vi "IMAQdx Acquisition Template (Host)-test.vi"() -> ()   [LabVIEW 2016]
uses:
  <vilib>/userdefined/High Color/IMAQdx.ctl
  <vilib>/vision/driver/IMAQdx.llb/IMAQdx Acquisition Mode.ctl
  <vilib>/vision/driver/IMAQdx.llb/IMAQdx Buffer Number Mode.ctl
  <vilib>/FPGAPlugInAG/roboRIO/niLvFpga_Open_roboRIO.vi
  <vilib>/rvi/interface/common/dynamic/niFpgaDynamicAddResources.vi
  <vilib>/FPGAPlugInAG/Dynamic/niLvFpga_Download_Dynamic.vi
  <vilib>/FPGAPlugInAG/Dynamic/niLvFpga_Run_Dynamic.vi
  <vilib>/visionFPGA/Basics/Configure Image Transfer to Target/IMAQ FPGA Configure Image Transfer to Target U32.vi
  <vilib>/Utility/error.llb/Error Cluster From Error Code.vi
  <vilib>/rvi/errors/niLvFpgaAdjustHostInterfaceError.vi
  <vilib>/visionFPGA/Basics/Image Transfer to Target/IMAQ FPGA Image Transfer to Target U32.vi
  <vilib>/rvi/interface/common/niFpgaWaitOnOcc.vi
  <vilib>/FPGAPlugInAG/Dynamic/niLvFpga_Close_Dynamic.vi
  <vilib>/rvi/interface/nirviOpenFPGA/nirviOpenFPGA.xnode
  FPGA Bitfiles/ImageProcessingw_FPGATarget2_ImageProcessingw_ZcF2hsHpmf8.lvbitx
  <vilib>/rvi/interface/nirviMethod/nirviMethod.xnode
  <vilib>/rvi/interface/nirviReadWriteControl/nirviReadWriteControl.xnode
  <vilib>/rvi/interface/nirviCloseFPGA/nirviCloseFPGA.xnode
  <vilib>/vision/driver/NI_Vision_Acquisition_Software.lvlib
  <resource>/objmgr/imaqdx.rc
  <vilib>/visionFPGA/NI_VDM_FPGA_Basics.lvlib
  <vilib>/rvi/interface/Simulation/niFpgaSimulationCallBeginRW.vi
  <vilib>/rvi/errors/niLvFpgaMergeErrorWithErrorCode.vi
  <vilib>/FPGAPlugInAG/Dynamic/niLvFpga_ReadFifo_Dynamic.vi
  <vilib>/FPGAPlugInAG/Dynamic/niLvFpga_ConfigureFifo_Dynamic.vi
  <vilib>/FPGAPlugInAG/Dynamic/niLvFpga_StartFifo_Dynamic.vi
  NiFpgaLv.dll
panel:
  out "OriImage Err out":errorcluster
  out "Image":T1(plugin-control)
  out "Count":i32
  out "error out 2":errorcluster
  in  "Camera":T2
  out "Error Out":errorcluster
  in  "Stop":bool
  # "Overview: Demonstrates how to acquire an image from a camera using the IMAQdx API, transfer the image to a FPGA target for processing, and retrieve the processed image for display or further processing on the host.\nRequirements:\n- LabVIEW FPGA\n- Vision Acquisition Software\n- Vision Development Module\nInstructions:\n1. Select a Camera\n2. Run the VI."
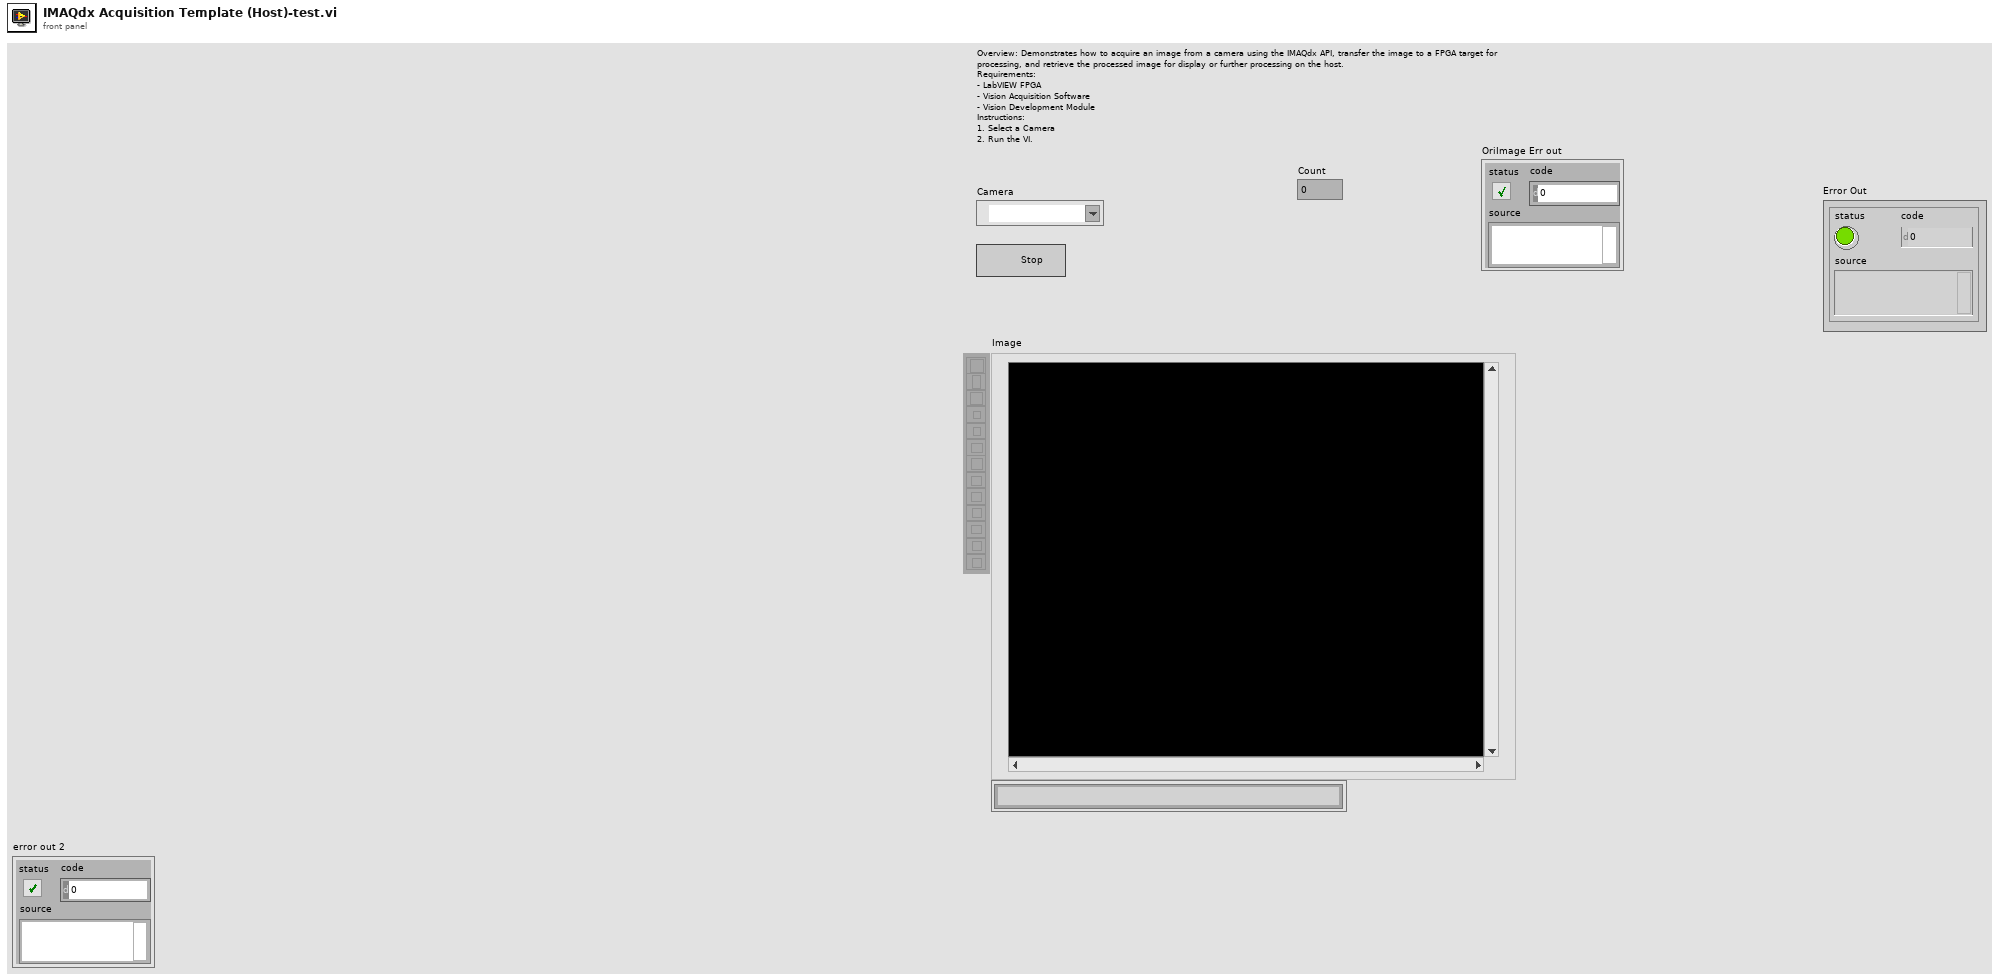
[diagram p1: front panel]
types:
  T1 = typedef "IMAQ Image.ctl" = refnum<image>
  T2 = typedef "IMAQdx.ctl" = refnum<k21>
  T3 = typedef "Image Type" = u32
  T4 = typedef "NI_Vision_Acquisition_Software.lvlib/IMAQdx Acquisition Mode.ctl" = enum32{"One Shot", "Continuous"}
  T5 = typedef "NI_Vision_Acquisition_Software.lvlib/IMAQdx Buffer Number Mode.ctl" = enum32{"Next", "Last", "Buffer Number", "Every", "Last New"}
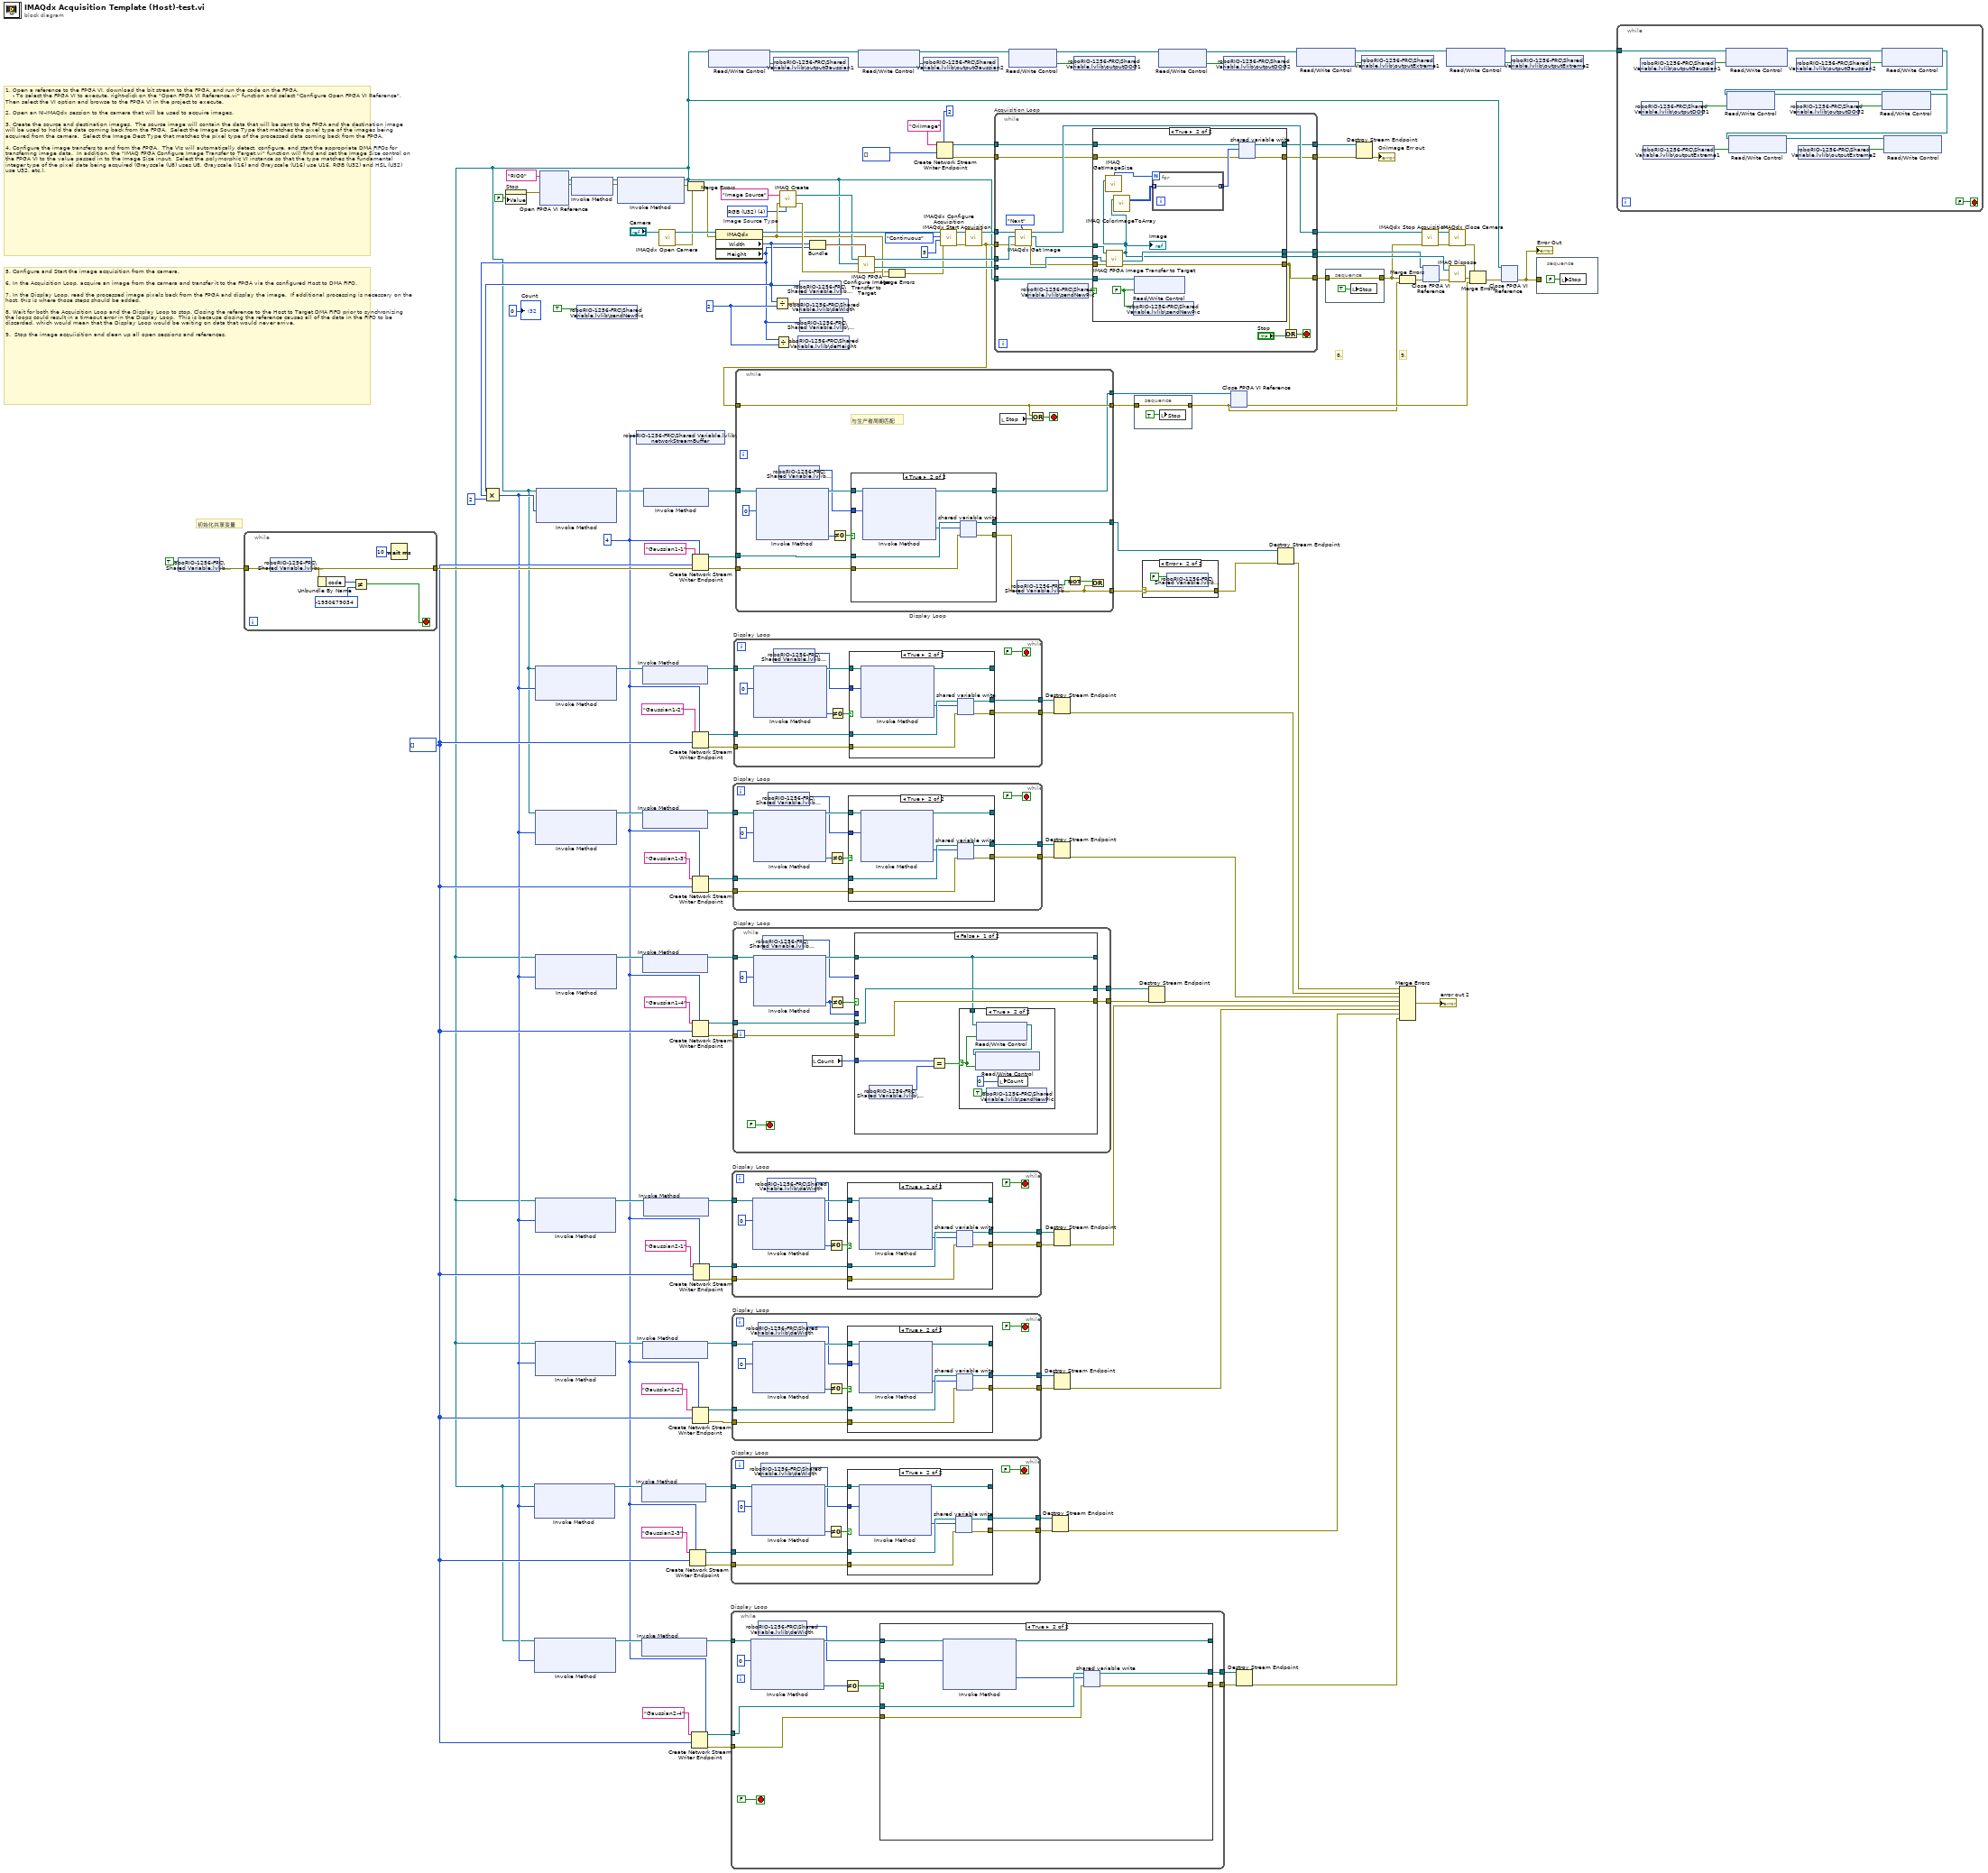
[diagram p0: block diagram]
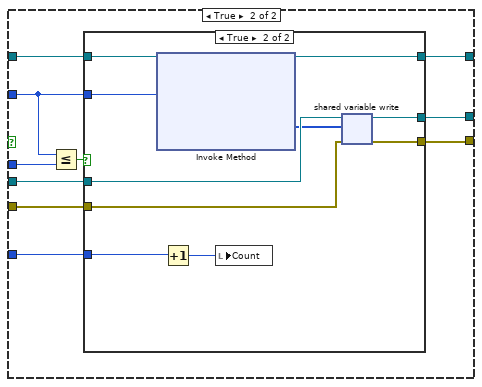
[diagram p6: hidden frame]
diagram:
  w16 = u32 2 ("y")
  w28 = i32[] []
  w25 = 4 ("writer buffer size")
  w110 = T3 4 items=["Grayscale (U8)", "Grayscale (I16)", "Grayscale (SGL)", "Complex (CSG)", "RGB (U32)", "HSL (U32)", "RGB (U64)", "Grayscale (U16)"]  # Image Source Type
  # "初始化共享变量"
  # "5. Configure and Start the image acquisition from the camera.\n\n6. In the Acquisition Loop, acquire an image from the camera and transfer it to the FPGA via the configured Host to DMA FIFO.\n\n7. In the Display Loop, read the processed image pixels back from the FPGA and display the image.  If additional processing is necessary on the host, this is where those steps should be added.\n\n8. Wait for both the Acquisition Loop and the Display Loop to stop. Closing the reference to the Host to Target DMA FIFO prior to synchronizing the loops could result in a timeout error in the Display Loop.  This is because closing the reference causes all of the data in the FIFO to be discarded, which would mean that the Display Loop would be waiting on data that would never arrive.\n\n9.  Stop the image acquiisition and clean up all open sessions and references."
  # "1. Open a reference to the FPGA VI, download the bit stream to the FPGA, and run the code on the FPGA.\n    - To select the FPGA VI to execute, right-click on the \"Open FPGA VI Reference.vi\" function and select \"Configure Open FPGA VI Reference\".  Then select the VI option and browse to the FPGA VI in the project to execute.\n\n2. Open an NI-IMAQdx session to the camera that will be used to acquire images.\n\n3. Create the source and destination images.  The source image will contain the data that will be sent to the FPGA and the destination image will be used to hold the data coming back from the FPGA.  Select the Image Source Type that matches the pixel type of the images being acquired from the camera.  Select the Image Dest Type that matches the pixel type of the processed data coming back from the FPGA.\n\n4. Configure the image transfers to and from the FPGA.  The VIs will automatically detect, configure, and start the appropriate DMA FIFOs for transferring image data.  In addition, the \"IMAQ FPGA Configure Image Transfer to Target.vi\" function will find and set the Image Size control on the FPGA VI to the value passed in to the Image Size input.  Select the polymorphic VI instance so that the type matches the fundamental integer type of the pixel data being acquired (Grayscale (U8) uses U8, Grayscale (I16) and Grayscale (U16) use U16, RGB (U32) and HSL (U32) use U32, etc.)."
  # "9."
  # "8."
  n1 = shared-variable "roboRIO-1256-FRC\\Shared Variable.lvlib\\Active"(TRUE ("Active?")) -> (error out=w96:errorcluster)  [unwired: 1 in]
  n2 = while {
    tunnel: w96 -> [w153]
    tunnel: [w150] -> w95
    stop <- w149 stop-if-true
    n3 = shared-variable "roboRIO-1256-FRC\\Shared Variable.lvlib\\Active"(error in=w153) -> (error out=w150:errorcluster)  [unwired: 1 out]
    n4 = Unbundle By Name(w150) -> ("code"=w152:i32)
    n5 = Not Equal?(x=w152, y=-1950679034) -> (x != y?=w149:bool)
    n6 = Wait (ms)(milliseconds to wait=u32 10) -> ()  [unwired: 1 out]
  }
  n7 = property on="Stop" class="Bool (strict)"("Value"=FALSE ("Stop")) -> (error out=w145:errorcluster)  [unwired: 2 in, 1 out]
  n8 = xnode "Open FPGA VI Reference"("error in"=w145, "resource name"=tag "RIO0") -> ("FPGA VI Reference Out"=w141:refnum<k20>, "error out"=w142:errorcluster)
  n9 = xnode "Invoke Method"("FPGA VI Reference In"=w141, "error in"=w142) -> ("FPGA VI Reference Out"=w144:refnum<k20>, "error out"=w143:errorcluster)
  n10 = shared-variable "roboRIO-1256-FRC\\Shared Variable.lvlib\\sendNewPic"(TRUE) -> ()  [unwired: 1 in, 1 out]
  n11 = xnode "Invoke Method"("FPGA VI Reference In"=w144, "error in"=w143) -> ("FPGA VI Reference Out"=w2:refnum<k20>, "error out"=w130:errorcluster)  [unwired: 1 in]
  n12 = shared-variable "roboRIO-1256-FRC\\Shared Variable.lvlib\\networkStreamBuffer"(w25) -> ()  [unwired: 1 in, 1 out]
  n13 = call <vilib>:"IMAQdx Open Camera.vi"("Session In"="Camera") -> ("error out"=w115:errorcluster, "Session Out"=w116:T2)  [unwired: 9 in]
  n14 = Merge Errors(w130, w115) -> (w114:errorcluster)
  n15 = Create Network Stream Writer Endpoint(7:w25, 9:w28, 11:"Gaussian2-3" ("writer name")) -> (0:w32:errorcluster, 3:w31:refnum<k21>)  [unwired: 4 in]
  n16 = Create Network Stream Writer Endpoint(7:w25, 9:w28, 11:"Gaussian2-4" ("writer name")) -> (0:w57:errorcluster, 3:w58:refnum<k21>)  [unwired: 4 in]
  n17 = Create Network Stream Writer Endpoint(7:w25, 9:w28, 11:"Gaussian2-2" ("writer name")) -> (0:w39:errorcluster, 3:w40:refnum<k21>)  [unwired: 4 in]
  n18 = Create Network Stream Writer Endpoint(7:w25, 8:w95, 9:w28, 11:"Gaussian1-1" ("writer name")) -> (0:w91:errorcluster, 3:w90:refnum<k21>)  [unwired: 3 in]
  n19 = Create Network Stream Writer Endpoint(7:w25, 9:w28, 11:"Gaussian1-2" ("writer name")) -> (0:w72:errorcluster, 3:w73:refnum<k21>)  [unwired: 4 in]
  n20 = Create Network Stream Writer Endpoint(7:w25, 9:w28, 11:"Gaussian1-3" ("writer name")) -> (0:w67:errorcluster, 3:w66:refnum<k21>)  [unwired: 4 in]
  n21 = Create Network Stream Writer Endpoint(7:w25, 9:w28, 11:"Gaussian1-4" ("writer name")) -> (0:w51:errorcluster, 3:w52:refnum<k21>)  [unwired: 4 in]
  n22 = Create Network Stream Writer Endpoint(7:w25, 9:w28, 11:"Gaussian2-1" ("writer name")) -> (0:w46:errorcluster, 3:w45:refnum<k21>)  [unwired: 4 in]
  n23 = xnode "Read/Write Control"("FPGA VI Reference In"=w2) -> ("FPGA VI Reference Out"=w11:refnum<k20>, "outputGaussian1"=w13:bool)  [unwired: 1 in, 1 out]
  n24 = property class="IMAQdx"(reference=w116, error in=w114) -> (reference out=w123:T2, error out=w111:errorcluster, "Width"=w18:u32, "Height"=w15:u32)
  n25 = Compound Arithmetic op=MULTIPLY(w18, w15, u32 2 ("value")) -> (w24:u32)
  n26 = xnode "Invoke Method"("FPGA VI Reference In"=w2, "Requested Depth"=w24) -> ("FPGA VI Reference Out"=w33:refnum<k20>)  [unwired: 1 in, 2 out]
  n27 = xnode "Invoke Method"("FPGA VI Reference In"=w2, "Requested Depth"=w24) -> ("FPGA VI Reference Out"=w56:refnum<k20>)  [unwired: 1 in, 2 out]
  n28 = xnode "Invoke Method"("FPGA VI Reference In"=w2, "Requested Depth"=w24) -> ("FPGA VI Reference Out"=w27:refnum<k20>)  [unwired: 1 in, 2 out]
  n29 = xnode "Invoke Method"("FPGA VI Reference In"=w2, "Requested Depth"=w24) -> ("FPGA VI Reference Out"=w38:refnum<k20>)  [unwired: 1 in, 2 out]
  n30 = xnode "Invoke Method"("FPGA VI Reference In"=w2, "Requested Depth"=w24) -> ("FPGA VI Reference Out"=w71:refnum<k20>)  [unwired: 1 in, 2 out]
  n31 = xnode "Invoke Method"("FPGA VI Reference In"=w2, "Requested Depth"=w24) -> ("FPGA VI Reference Out"=w68:refnum<k20>)  [unwired: 1 in, 2 out]
  n32 = xnode "Invoke Method"("FPGA VI Reference In"=w2, "Requested Depth"=w24) -> ("FPGA VI Reference Out"=w50:refnum<k20>)  [unwired: 1 in, 2 out]
  n33 = xnode "Invoke Method"("FPGA VI Reference In"=w2, "Requested Depth"=w24) -> ("FPGA VI Reference Out"=w100:refnum<k20>)  [unwired: 1 in, 2 out]
  n34 = xnode "Invoke Method"("FPGA VI Reference In"=w33) -> ("FPGA VI Reference Out"=w34:refnum<k20>)  [unwired: 1 in, 1 out]
  n35 = xnode "Invoke Method"("FPGA VI Reference In"=w56) -> ("FPGA VI Reference Out"=w55:refnum<k20>)  [unwired: 1 in, 1 out]
  n36 = xnode "Invoke Method"("FPGA VI Reference In"=w38) -> ("FPGA VI Reference Out"=w37:refnum<k20>)  [unwired: 1 in, 1 out]
  n37 = xnode "Invoke Method"("FPGA VI Reference In"=w71) -> ("FPGA VI Reference Out"=w70:refnum<k20>)  [unwired: 1 in, 1 out]
  n38 = xnode "Invoke Method"("FPGA VI Reference In"=w68) -> ("FPGA VI Reference Out"=w69:refnum<k20>)  [unwired: 1 in, 1 out]
  n39 = xnode "Invoke Method"("FPGA VI Reference In"=w50) -> ("FPGA VI Reference Out"=w49:refnum<k20>)  [unwired: 1 in, 1 out]
  n40 = xnode "Invoke Method"("FPGA VI Reference In"=w100) -> ("FPGA VI Reference Out"=w99:refnum<k20>)  [unwired: 1 in, 1 out]
  n41 = xnode "Invoke Method"("FPGA VI Reference In"=w27) -> ("FPGA VI Reference Out"=w26:refnum<k20>)  [unwired: 1 in, 1 out]
  n42 = while "Display Loop" {
    tunnel: [w164] -> w61
    tunnel: w57 -> [w163]
    tunnel: w58 -> [w162]
    tunnel: [w157] -> w60
    tunnel: w55 -> [w156]
    stop <- FALSE stop-if-true
    n43 = xnode "Invoke Method"("FPGA VI Reference In"=w156, "Number of Elements"=u32 0) -> ("FPGA VI Reference Out"=w159:refnum<k20>, "Elements Remaining"=w154:u32)  [unwired: 2 in, 2 out]
    n44 = shared-variable "roboRIO-1256-FRC\\Shared Variable.lvlib\\deWidth"() -> (w155:u16)  [unwired: 1 in, 1 out]
    n45 = Not Equal To 0?(x=w154) -> (x != 0?=w161:bool)
    n46 = case shown="True" w161 {
      tunnel: w159 -> [w165 w175]
      tunnel: [w167 w174] -> w164
      tunnel: w163 -> [w166 w173]
      tunnel: w162 -> [w167 w172]
      tunnel: [w166 w171] -> w157
      tunnel: [w165 w170] -> _
      tunnel: w155 -> [_ w169]
      frame False {
      }
      frame True {
        n47 = xnode "Invoke Method"("FPGA VI Reference In"=w175, "Number of Elements"=w169) -> ("FPGA VI Reference Out"=w170:refnum<k20>, "Data"=w168:u8[])  [unwired: 2 in, 2 out]
        n48 = shared-variable-write(w172, w173, w168) -> (w174:refnum<k21>, w171:errorcluster)  [unwired: 1 in, 1 out]
      }
    }
  }
  n49 = while "Display Loop" {
    tunnel: [w186] -> w29
    tunnel: w32 -> [w185]
    tunnel: w31 -> [w184]
    tunnel: [w178] -> w30
    tunnel: w34 -> [w177]
    stop <- FALSE stop-if-true
    (unwired) u32 640 ("Number of Elements")
    n50 = xnode "Invoke Method"("FPGA VI Reference In"=w177, "Number of Elements"=u32 0) -> ("FPGA VI Reference Out"=w180:refnum<k20>, "Elements Remaining"=w181:u32)  [unwired: 2 in, 2 out]
    n51 = shared-variable "roboRIO-1256-FRC\\Shared Variable.lvlib\\deWidth"() -> (w176:u16)  [unwired: 1 in, 1 out]
    n52 = Not Equal To 0?(x=w181) -> (x != 0?=w183:bool)
    n53 = case shown="True" w183 {
      tunnel: w180 -> [w187 w197]
      tunnel: [w189 w196] -> w186
      tunnel: w185 -> [w188 w195]
      tunnel: w184 -> [w189 w194]
      tunnel: [w188 w193] -> w178
      tunnel: [w187 w191] -> _
      tunnel: w176 -> [_ w190]
      frame False {
      }
      frame True {
        n54 = xnode "Invoke Method"("FPGA VI Reference In"=w197, "Number of Elements"=w190) -> ("FPGA VI Reference Out"=w191:refnum<k20>, "Data"=w192:u8[])  [unwired: 2 in, 2 out]
        n55 = shared-variable-write(w194, w195, w192) -> (w196:refnum<k21>, w193:errorcluster)  [unwired: 1 in, 1 out]
      }
    }
  }
  n56 = while "Display Loop" {
    tunnel: [w208] -> w43
    tunnel: w46 -> [w207]
    tunnel: w45 -> [w206]
    tunnel: [w200] -> w44
    tunnel: w26 -> [w199]
    stop <- FALSE stop-if-true
    (unwired) u32 640 ("Number of Elements")
    n57 = xnode "Invoke Method"("FPGA VI Reference In"=w199, "Number of Elements"=u32 0) -> ("FPGA VI Reference Out"=w202:refnum<k20>, "Elements Remaining"=w203:u32)  [unwired: 2 in, 2 out]
    n58 = shared-variable "roboRIO-1256-FRC\\Shared Variable.lvlib\\deWidth"() -> (w198:u16)  [unwired: 1 in, 1 out]
    n59 = Not Equal To 0?(x=w203) -> (x != 0?=w205:bool)
    n60 = case shown="True" w205 {
      tunnel: w202 -> [w209 w219]
      tunnel: [w211 w218] -> w208
      tunnel: w207 -> [w210 w217]
      tunnel: w206 -> [w211 w216]
      tunnel: [w210 w215] -> w200
      tunnel: [w209 w213] -> _
      tunnel: w198 -> [_ w212]
      frame False {
      }
      frame True {
        n61 = xnode "Invoke Method"("FPGA VI Reference In"=w219, "Number of Elements"=w212) -> ("FPGA VI Reference Out"=w213:refnum<k20>, "Data"=w214:u8[])  [unwired: 2 in, 2 out]
        n62 = shared-variable-write(w216, w217, w214) -> (w218:refnum<k21>, w215:errorcluster)  [unwired: 1 in, 1 out]
      }
    }
  }
  n63 = while "Display Loop" {
    tunnel: [w230] -> w42
    tunnel: w39 -> [w229]
    tunnel: w40 -> [w228]
    tunnel: [w222] -> w41
    tunnel: w37 -> [w221]
    stop <- FALSE stop-if-true
    (unwired) u32 640 ("Number of Elements")
    n64 = xnode "Invoke Method"("FPGA VI Reference In"=w221, "Number of Elements"=u32 0) -> ("FPGA VI Reference Out"=w224:refnum<k20>, "Elements Remaining"=w225:u32)  [unwired: 2 in, 2 out]
    n65 = shared-variable "roboRIO-1256-FRC\\Shared Variable.lvlib\\deWidth"() -> (w220:u16)  [unwired: 1 in, 1 out]
    n66 = Not Equal To 0?(x=w225) -> (x != 0?=w227:bool)
    n67 = case shown="True" w227 {
      tunnel: w224 -> [w231 w241]
      tunnel: [w233 w240] -> w230
      tunnel: w229 -> [w232 w239]
      tunnel: w228 -> [w233 w238]
      tunnel: [w232 w237] -> w222
      tunnel: [w231 w235] -> _
      tunnel: w220 -> [_ w234]
      frame False {
      }
      frame True {
        n68 = xnode "Invoke Method"("FPGA VI Reference In"=w241, "Number of Elements"=w234) -> ("FPGA VI Reference Out"=w235:refnum<k20>, "Data"=w236:u8[])  [unwired: 2 in, 2 out]
        n69 = shared-variable-write(w238, w239, w236) -> (w240:refnum<k21>, w237:errorcluster)  [unwired: 1 in, 1 out]
      }
    }
  }
  n70 = while "Display Loop" {
    tunnel: [w252] -> w63
    tunnel: w67 -> [w251]
    tunnel: w66 -> [w250]
    tunnel: [w244] -> w64
    tunnel: w69 -> [w243]
    stop <- FALSE stop-if-true
    (unwired) u32 640 ("Number of Elements")
    n71 = xnode "Invoke Method"("FPGA VI Reference In"=w243, "Number of Elements"=u32 0) -> ("FPGA VI Reference Out"=w246:refnum<k20>, "Elements Remaining"=w247:u32)  [unwired: 2 in, 2 out]
    n72 = shared-variable "roboRIO-1256-FRC\\Shared Variable.lvlib\\Width"() -> (w242:u16)  [unwired: 1 in, 1 out]
    n73 = Not Equal To 0?(x=w247) -> (x != 0?=w249:bool)
    n74 = case shown="True" w249 {
      tunnel: w246 -> [w253 w263]
      tunnel: [w255 w262] -> w252
      tunnel: w251 -> [w254 w261]
      tunnel: w250 -> [w255 w260]
      tunnel: [w254 w259] -> w244
      tunnel: [w253 w257] -> _
      tunnel: w242 -> [_ w256]
      frame False {
      }
      frame True {
        n75 = xnode "Invoke Method"("FPGA VI Reference In"=w263, "Number of Elements"=w256) -> ("FPGA VI Reference Out"=w257:refnum<k20>, "Data"=w258:u8[])  [unwired: 2 in, 2 out]
        n76 = shared-variable-write(w260, w261, w258) -> (w262:refnum<k21>, w259:errorcluster)  [unwired: 1 in, 1 out]
      }
    }
  }
  n77 = while "Display Loop" {
    tunnel: [w275] -> w54
    tunnel: w51 -> [w274]
    tunnel: w52 -> [w273]
    tunnel: [w268] -> w53
    tunnel: w49 -> [w267]
    stop <- FALSE stop-if-true
    n78 = xnode "Invoke Method"("FPGA VI Reference In"=w267, "Number of Elements"=u32 0) -> ("FPGA VI Reference Out"=w270:refnum<k20>, "Elements Remaining"=w264:u32)  [unwired: 2 in, 2 out]
    n79 = shared-variable "roboRIO-1256-FRC\\Shared Variable.lvlib\\Width"() -> (w266:u16)  [unwired: 1 in, 1 out]
    n80 = local read "Count"() -> (w265:i32)
    n81 = Not Equal To 0?(x=w264) -> (x != 0?=w272:bool)
    n82 = case shown="False" w272 {
      tunnel: w270 -> [w276 w296]
      tunnel: [w281 w295] -> w275
      tunnel: w274 -> [w280 w294]
      tunnel: w273 -> [w281 w293]
      tunnel: [w280 w292] -> w268
      tunnel: [w276 w291] -> _
      tunnel: w266 -> [_ w288]
      tunnel: w265 -> [w278 w290]
      tunnel: w264 -> [_ w287]
      frame False {
        n83 = shared-variable "roboRIO-1256-FRC\\Shared Variable.lvlib\\Height"() -> (w277:u16)  [unwired: 1 in, 1 out]
        n84 = Equal?(x=w278, y=w277) -> (x = y?=w279:bool)
        n85 = case shown="True" w279 {
          selector: w279 -> [_ w283]
          tunnel: w276 -> [_ w286]
          frame False {
          }
          frame True {
            n86 = xnode "Read/Write Control"("FPGA VI Reference In"=w286, "StartOfImage"=w283) -> ("FPGA VI Reference Out"=w285:refnum<k20>)  [unwired: 1 in, 1 out]
            n87 = xnode "Read/Write Control"("FPGA VI Reference In"=w285, "Ready For Output"=w283) -> ()  [unwired: 1 in, 2 out]
            n88 = shared-variable "roboRIO-1256-FRC\\Shared Variable.lvlib\\sendNewPic"(TRUE ("sendNewPic")) -> ()  [unwired: 1 in, 1 out]
            n89 = local write "Count"(0) -> ()
          }
        }
      }
      frame True {
        n90 = Less Or Equal?(x=w288, y=w287) -> (x <= y?=w289:bool)
        n91 = case shown="True" w289 {
          tunnel: w296 -> [w299 w309]
          tunnel: [w298 w308] -> w295
          tunnel: w294 -> [w297 w307]
          tunnel: w293 -> [w298 w306]
          tunnel: [w297 w305] -> w292
          tunnel: [w299 w303] -> w291
          tunnel: w288 -> [_ w302]
          tunnel: w290 -> [_ w301]
          frame False {
          }
          frame True {
            n92 = xnode "Invoke Method"("FPGA VI Reference In"=w309, "Number of Elements"=w302) -> ("FPGA VI Reference Out"=w303:refnum<k20>, "Data"=w304:u8[])  [unwired: 2 in, 2 out]
            n93 = Increment(x=w301) -> (x+1=w300:i32)
            n94 = local write "Count"(w300) -> ()
            n95 = shared-variable-write(w306, w307, w304) -> (w308:refnum<k21>, w305:errorcluster)  [unwired: 1 in, 1 out]
          }
        }
      }
    }
  }
  n96 = while "Display Loop" {
    tunnel: [w320] -> w80
    tunnel: w72 -> [w319]
    tunnel: w73 -> [w318]
    tunnel: [w312] -> w79
    tunnel: w70 -> [w311]
    stop <- FALSE stop-if-true
    (unwired) u32 640 ("Number of Elements")
    n97 = xnode "Invoke Method"("FPGA VI Reference In"=w311, "Number of Elements"=u32 0) -> ("FPGA VI Reference Out"=w314:refnum<k20>, "Elements Remaining"=w315:u32)  [unwired: 2 in, 2 out]
    n98 = shared-variable "roboRIO-1256-FRC\\Shared Variable.lvlib\\Width"() -> (w310:u16)  [unwired: 1 in, 1 out]
    n99 = Not Equal To 0?(x=w315) -> (x != 0?=w317:bool)
    n100 = case shown="True" w317 {
      tunnel: w314 -> [w321 w331]
      tunnel: [w323 w330] -> w320
      tunnel: w319 -> [w322 w329]
      tunnel: w318 -> [w323 w328]
      tunnel: [w322 w327] -> w312
      tunnel: [w321 w325] -> _
      tunnel: w310 -> [_ w324]
      frame False {
      }
      frame True {
        n101 = xnode "Invoke Method"("FPGA VI Reference In"=w331, "Number of Elements"=w324) -> ("FPGA VI Reference Out"=w325:refnum<k20>, "Data"=w326:u8[])  [unwired: 2 in, 2 out]
        n102 = shared-variable-write(w328, w329, w326) -> (w330:refnum<k21>, w327:errorcluster)  [unwired: 1 in, 1 out]
      }
    }
  }
  n103 = shared-variable "roboRIO-1256-FRC\\Shared Variable.lvlib\\outputGaussian1"(w13) -> ()  [unwired: 1 in, 1 out]
  n104 = Divide(x=w18, y=w16) -> (x/y=w17:dbl)
  n105 = Divide(x=w15, y=w16) -> (x/y=w14:dbl)
  n106 = call "IMAQ Create"("Image Name"="Image Source", "Image Type"=w110, "error in (no error)"=w111) -> ("New Image"=w121:T1, "error out"=w129:errorcluster)  [unwired: 2 in]
  n107 = shared-variable "roboRIO-1256-FRC\\Shared Variable.lvlib\\deHeight"(w14) -> ()  [unwired: 1 in, 1 out]
  n108 = shared-variable "roboRIO-1256-FRC\\Shared Variable.lvlib\\Width"(w18) -> ()  [unwired: 1 in, 1 out]
  n109 = shared-variable "roboRIO-1256-FRC\\Shared Variable.lvlib\\deWidth"(w17) -> ()  [unwired: 1 in, 1 out]
  n110 = shared-variable "roboRIO-1256-FRC\\Shared Variable.lvlib\\Height"(w15) -> ()  [unwired: 1 in, 1 out]
  n111 = Bundle("Width"=w18, "Height"=w15) -> (w128:cluster{"Width":u32, "Height":u32})  [unwired: 1 in]
  n112 = xnode "Read/Write Control"("FPGA VI Reference In"=w11) -> ("FPGA VI Reference Out"=w7:refnum<k20>, "outputGaussian2"=w12:bool)  [unwired: 1 in, 1 out]
  n113 = call-poly <vilib>:"IMAQ FPGA Configure Image Transfer to Target.vi"("Image Size"=w128, "error in (no error)"=w129, "FPGA VI Reference In"=w2, "Image"=w121) -> ("error out"=w104:errorcluster, "DMA FIFO Reference Out"=w139:refnum<k20>, "Image Out"=w140:T1)  [unwired: 4 in, 1 out]
  n114 = Merge Errors(w104, w111) -> (w103:errorcluster)
  n115 = shared-variable "roboRIO-1256-FRC\\Shared Variable.lvlib\\outputGaussian2"(w12) -> ()  [unwired: 1 in, 1 out]
  n116 = Create Network Stream Writer Endpoint(7:2 ("writer buffer size"), 9:i32[] [], 11:"OriImage" ("writer name")) -> (0:w84:errorcluster, 3:w85:refnum<k21>)  [unwired: 4 in]
  n117 = call <vilib>:"IMAQdx Configure Acquisition.vi"("error in"=w103, "Number of Buffers"=u32 5, "Continuous?"=IMAQdx_Acquisition_Mode."Continuous", "Session In"=w123) -> ("error out"=w126:errorcluster, "Session Out"=w127:T2)  [unwired: 6 in]
  n118 = call <vilib>:"IMAQdx Start Acquisition.vi"("error in"=w126, "Session In"=w127) -> ("error out"=w102:errorcluster, "Session Out"=w122:T2)  [unwired: 8 in]
  n119 = while "Display Loop" {
    tunnel: w102 -> [w347]
    tunnel: [w335] -> w136
    tunnel: [w347] -> w135
    tunnel: w99 -> [w336]
    tunnel: [w345] -> w93
    tunnel: [w344] -> w92
    tunnel: w91 -> [w343]
    tunnel: w90 -> [w342]
    stop <- w348 stop-if-true
    (unwired) u32 640 ("Number of Elements")
    # "与生产者周期匹配"
    n120 = xnode "Invoke Method"("FPGA VI Reference In"=w336, "Number of Elements"=u32 0) -> ("FPGA VI Reference Out"=w333:refnum<k20>, "Elements Remaining"=w334:u32)  [unwired: 2 in, 2 out]
    n121 = shared-variable "roboRIO-1256-FRC\\Shared Variable.lvlib\\Width"() -> (w332:u16)  [unwired: 1 in, 1 out]
    n122 = Not Equal To 0?(x=w334) -> (x != 0?=w338:bool)
    n123 = case shown="True" w338 {
      tunnel: w333 -> [w349 w359]
      tunnel: [w351 w358] -> w344
      tunnel: w343 -> [w350 w357]
      tunnel: w342 -> [w351 w356]
      tunnel: [w350 w355] -> w341
      tunnel: [w349 w353] -> w335
      tunnel: w332 -> [_ w352]
      frame False {
      }
      frame True {
        n124 = xnode "Invoke Method"("FPGA VI Reference In"=w359, "Number of Elements"=w352) -> ("FPGA VI Reference Out"=w353:refnum<k20>, "Data"=w354:u8[])  [unwired: 2 in, 2 out]
        n125 = shared-variable-write(w356, w357, w354) -> (w358:refnum<k21>, w355:errorcluster)  [unwired: 1 in, 1 out]
      }
    }
    n126 = local read "Stop"() -> (w346:bool)
    n127 = shared-variable "roboRIO-1256-FRC\\Shared Variable.lvlib\\Active"(error in=w341) -> (w339:bool, error out=w345:errorcluster)
    n128 = Or(x=w347, y=w346) -> (x .or. y?=w348:bool)
    n129 = Not(x=w339) -> (.not. x?=w340:bool)
    n130 = Or(x=w340, y=w345) -> ()  [unwired: 1 out]
  }
  n131 = while "Acquisition Loop" {
    tunnel: [w369] -> w108
    tunnel: w140 -> [w374]
    tunnel: w139 -> [w371]
    tunnel: [w370] -> w109
    tunnel: [w367] -> w138
    tunnel: w122 -> [w375]
    tunnel: [w373] -> w118
    tunnel: w102 -> [w372]
    tunnel: w2 -> [w365]
    tunnel: w85 -> [w364]
    tunnel: w84 -> [w363]
    tunnel: [w362] -> w83
    tunnel: [w361] -> w82
    stop <- w377 stop-if-true
    n132 = call <vilib>:"IMAQdx Get Image.vi"("Buffer Number Mode (Next)"=IMAQdx_Buffer_Number_Mode."Next", "error in"=w372, "Image In"=w374, "Session In"=w375) -> ("error out"=w366:errorcluster, "Image Out"=w368:T1, "Session Out"=w373:T2)  [unwired: 4 in, 1 out]
    n133 = shared-variable "roboRIO-1256-FRC\\Shared Variable.lvlib\\sendNewPic"() -> (w360:bool)  [unwired: 1 in, 1 out]
    n134 = case shown="True" w360 {
      tunnel: w371 -> [w383 w398]
      tunnel: [w383 w394] -> w370
      tunnel: [w382 w395] -> w369
      tunnel: w368 -> [w381 w397]
      tunnel: [w381 w389] -> w367
      tunnel: w366 -> [w382 w396]
      tunnel: w365 -> [_ w392]
      tunnel: w364 -> [w380 w387]
      tunnel: w363 -> [w379 w386]
      tunnel: [w380 w385] -> w362
      tunnel: [w379 w384] -> w361
      frame False {
      }
      frame True {
        w393 = FALSE ("EndOfImage")
        n135 = call-poly <vilib>:"IMAQ FPGA Image Transfer to Target.vi"("error in (no error)"=w396, "DMA FIFO Reference In"=w398, "Image"=w397) -> ("error out"=w395:errorcluster, "DMA FIFO Reference Out"=w394:refnum<k20>, "Image Out"=w389:T1)  [unwired: 6 in]
        "Image" <- w389
        n136 = call "IMAQ GetImageSize"("Image"=w389) -> ("X Resolution"=w391:i32)  [unwired: 3 in, 2 out]
        n137 = call "IMAQ ColorImageToArray"("Image"=w389) -> ("Image Pixels (U32)"=w390:u32[][])  [unwired: 3 in, 2 out]
        n138 = shared-variable "roboRIO-1256-FRC\\Shared Variable.lvlib\\sendNewPic"(w393) -> ()  [unwired: 1 in, 1 out]
        n139 = xnode "Read/Write Control"("FPGA VI Reference In"=w392, "StartOfImage"=w393) -> ()  [unwired: 1 in, 2 out]
        n140 = for {
          N: w391 -> [_]
          tunnel: w390 -> [w399] mode=indexing
          tunnel: [w399] -> w388 mode=concatenating
        }
        n141 = shared-variable-write(w387, w386, w388) -> (w385:refnum<k21>, w384:errorcluster)  [unwired: 1 in, 1 out]
      }
    }
    n142 = Or(x=w369, y="Stop") -> (x .or. y?=w377:bool)
  }
  n143 = xnode "Read/Write Control"("FPGA VI Reference In"=w7) -> ("FPGA VI Reference Out"=w10:refnum<k20>, "outputDOG1"=w8:bool)  [unwired: 1 in, 1 out]
  n144 = Destroy Stream Endpoint(8:w30, 11:w29) -> (0:w20:errorcluster)
  n145 = Destroy Stream Endpoint(8:w41, 11:w42) -> (0:w21:errorcluster)
  n146 = Destroy Stream Endpoint(8:w79, 11:w80) -> (0:w75:errorcluster)
  n147 = Destroy Stream Endpoint(8:w64, 11:w63) -> (0:w62:errorcluster)
  n148 = Destroy Stream Endpoint(8:w44, 11:w43) -> (0:w22:errorcluster)
  n149 = shared-variable "roboRIO-1256-FRC\\Shared Variable.lvlib\\outputDOG1"(w8) -> ()  [unwired: 1 in, 1 out]
  n150 = stacked-sequence {
    tunnel: w135 -> [w400]
    tunnel: [w400] -> w107
    frame #0 {
      n151 = local write "Stop"(TRUE ("Stop")) -> ()
    }
  }
  n152 = case shown="Error" w93 {
    selector: w93 -> [w402 w403]
    tunnel: [w402 w403] -> w78
    frame No Error {
    }
    frame Error {
      n153 = shared-variable "roboRIO-1256-FRC\\Shared Variable.lvlib\\Active"(FALSE ("Active?")) -> ()  [unwired: 1 in, 1 out]
    }
  }
  n154 = Destroy Stream Endpoint(8:w53, 11:w54) -> (0:w23:errorcluster)
  n155 = xnode "Read/Write Control"("FPGA VI Reference In"=w10) -> ("FPGA VI Reference Out"=w3:refnum<k20>, "outputDOG2"=w9:bool)  [unwired: 1 in, 1 out]
  n156 = shared-variable "roboRIO-1256-FRC\\Shared Variable.lvlib\\outputDOG2"(w9) -> ()  [unwired: 1 in, 1 out]
  n157 = xnode "Close FPGA VI Reference"("FPGA VI Reference In"=w136, "error in"=w107) -> ("error out"=w134:errorcluster)
  n158 = Destroy Stream Endpoint(8:w60, 11:w61) -> (0:w19:errorcluster)
  n159 = Destroy Stream Endpoint(8:w78, 11:w92) -> (0:w76:errorcluster)
  n160 = xnode "Read/Write Control"("FPGA VI Reference In"=w3) -> ("FPGA VI Reference Out"=w4:refnum<k20>, "outputExtreme1"=w6:bool)  [unwired: 1 in, 1 out]
  n161 = stacked-sequence {
    tunnel: w108 -> [w405]
    tunnel: [w405] -> w105
    frame #0 {
      n162 = local write "Stop"(TRUE ("Stop")) -> ()
    }
  }
  n163 = Destroy Stream Endpoint(8:w82, 11:w83) -> (0:→"OriImage Err out":errorcluster)
  n164 = shared-variable "roboRIO-1256-FRC\\Shared Variable.lvlib\\outputExtreme1"(w6) -> ()  [unwired: 1 in, 1 out]
  n165 = Merge Errors(w105, w107) -> (w106:errorcluster)
  n166 = Merge Errors(w76, w75, w62, w23, w22, w21, w20, w19) -> (→"error out 2":errorcluster)
  n167 = call <vilib>:"IMAQdx Stop Acquisition.vi"("error in"=w105, "Session In"=w118) -> ("error out"=w119:errorcluster, "Session Out"=w120:T2)  [unwired: 8 in]
  n168 = xnode "Close FPGA VI Reference"("FPGA VI Reference In"=w109, "error in"=w106) -> ("error out"=w137:errorcluster)
  n169 = xnode "Read/Write Control"("FPGA VI Reference In"=w4) -> ("FPGA VI Reference Out"=w1:refnum<k20>, "outputExtreme2"=w5:bool)  [unwired: 1 in, 1 out]
  n170 = call <vilib>:"IMAQdx Close Camera.vi"("error in"=w119, "Session In"=w120) -> ("error out"=w117:errorcluster)  [unwired: 9 in]
  n171 = call "IMAQ Dispose"("Image"=w138, "error in (no error)"=w137) -> ("error out"=w133:errorcluster)  [unwired: 4 in]
  n172 = Merge Errors(w117, w133, w134) -> (w113:errorcluster)
  n173 = xnode "Close FPGA VI Reference"("FPGA VI Reference In"=w2, "error in"=w113) -> ("error out"=w112:errorcluster)
  "Error Out" <- w112
  n174 = shared-variable "roboRIO-1256-FRC\\Shared Variable.lvlib\\outputExtreme2"(w5) -> ()  [unwired: 1 in, 1 out]
  n175 = stacked-sequence {
    tunnel: w112 -> [_]
    frame #0 {
      n176 = local write "Stop"(FALSE ("Stop")) -> ()
    }
  }
  n177 = while {
    tunnel: w1 -> [w419]
    stop <- FALSE stop-if-true
    n178 = shared-variable "roboRIO-1256-FRC\\Shared Variable.lvlib\\outputGaussian1"() -> (w420:bool)  [unwired: 1 in, 1 out]
    n179 = shared-variable "roboRIO-1256-FRC\\Shared Variable.lvlib\\outputDOG1"() -> (w416:bool)  [unwired: 1 in, 1 out]
    n180 = shared-variable "roboRIO-1256-FRC\\Shared Variable.lvlib\\outputExtreme1"() -> (w410:bool)  [unwired: 1 in, 1 out]
    n181 = xnode "Read/Write Control"("FPGA VI Reference In"=w419, "outputGaussian1"=w420) -> ("FPGA VI Reference Out"=w418:refnum<k20>)  [unwired: 1 in, 1 out]
    n182 = shared-variable "roboRIO-1256-FRC\\Shared Variable.lvlib\\outputGaussian2"() -> (w417:bool)  [unwired: 1 in, 1 out]
    n183 = shared-variable "roboRIO-1256-FRC\\Shared Variable.lvlib\\outputDOG2"() -> (w414:bool)  [unwired: 1 in, 1 out]
    n184 = shared-variable "roboRIO-1256-FRC\\Shared Variable.lvlib\\outputExtreme2"() -> (w412:bool)  [unwired: 1 in, 1 out]
    n185 = xnode "Read/Write Control"("FPGA VI Reference In"=w418, "outputGaussian2"=w417) -> ("FPGA VI Reference Out"=w413:refnum<k20>)  [unwired: 1 in, 1 out]
    n186 = xnode "Read/Write Control"("FPGA VI Reference In"=w413, "outputDOG1"=w416) -> ("FPGA VI Reference Out"=w415:refnum<k20>)  [unwired: 1 in, 1 out]
    n187 = xnode "Read/Write Control"("FPGA VI Reference In"=w415, "outputDOG2"=w414) -> ("FPGA VI Reference Out"=w409:refnum<k20>)  [unwired: 1 in, 1 out]
    n188 = xnode "Read/Write Control"("FPGA VI Reference In"=w409, "outputExtreme1"=w410) -> ("FPGA VI Reference Out"=w411:refnum<k20>)  [unwired: 1 in, 1 out]
    n189 = xnode "Read/Write Control"("FPGA VI Reference In"=w411, "outputExtreme2"=w412) -> ()  [unwired: 1 in, 2 out]
  }
  "Count" <- 0
